vi "MPB_write_read_json text step array.vi"(8 "error in":errorcluster, 9 "json_array_from_file":T1[](array[typedef]) {"data num" format="%.3f"}, 10 "write_read":T3=enum."read", 11 "File Path":path) -> (0 "error out":errorcluster, 1 "steps array out":T1[](array[typedef]) {"data num" format="%.3f"}, 3 "File Path":path)   [LabVIEW 2020]
uses:
  controls/MPB_step.ctl
  controls/MPB_step_type.ctl
  controls/write_read.ctl
  3e47bdee-b09f-426d-96e8-78c270cf6aec.vi
  <vilib>/JDP Science/JSONtext/JSON text to Variant.vi
  <vilib>/JDP Science/JSONtext/JSONtext.lvlib
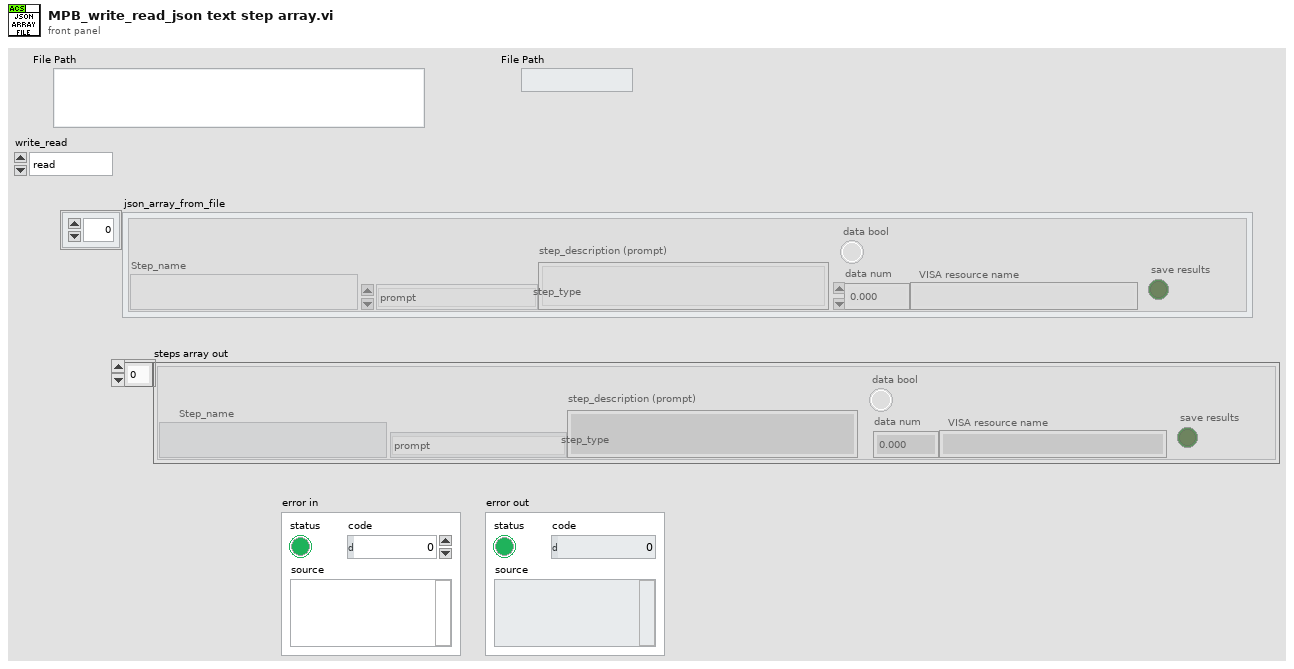
[diagram p1: front panel]
types:
  T1 = typedef "MPB_step.ctl" = cluster{"VISA resource name":string, "data num":dbl, "step_description (prompt)":string, "save results":bool, "step_type":T2, "Step_name":string, "data bool":bool}
  T2 = typedef "MPB_step_type.ctl" = enum16{"default", "prompt", "sequence#", "12V_1_power supply on_off", "12V_2_power supply on_off", "set_hipot_V", "set_hipot_I_limit", "set_hipot_ramping (sec)", "set hipot_hold_time", "read_hipot_V", "read_hipot_I", "set_daq", "read_daq", "flash uds", "wait (sec)", "record_pass_fail", "ac_charge_test", "dc_400V_charging", "HAPS Heater Output", "HAPS Compressor Output", "stop_test", "error_exit"}
  T3 = typedef "write_read.ctl" = enum16{"write", "read"}
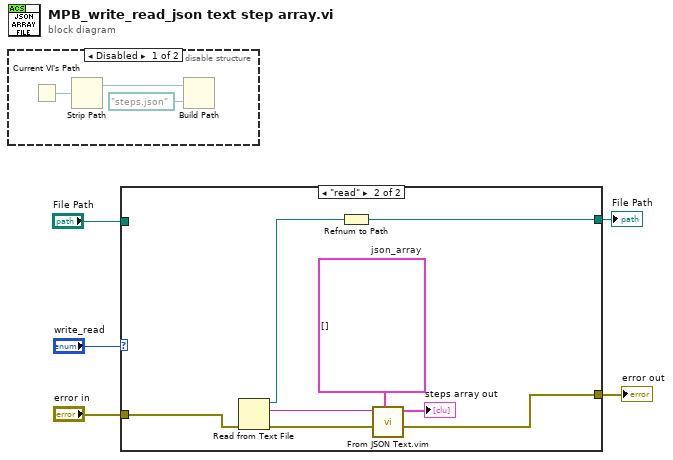
[diagram p0: block diagram]
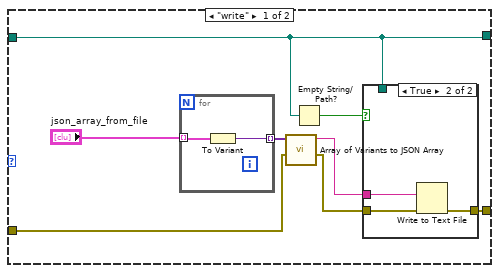
[diagram p3: hidden frame]
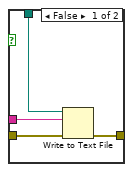
[diagram p4: hidden frame]
diagram:
  n1 = disable-structure shown="Disabled" {
    frame Disabled {
      n2 = Current VI's Path() -> (path=w8:path)
      n3 = Strip Path(path=w8) -> (stripped path=w7:path)  [unwired: 1 out]
      n4 = Build Path(base path=w7, name or relative path=path "steps.json") -> ()  [unwired: 1 out]
    }
    frame Enabled {
    }
  }
  n5 = case shown="\"read\"" "write_read" {
    tunnel: "error in" -> [w13 w30]
    tunnel: [w11 w28] -> w3
    tunnel: [w9 w26] -> w2
    tunnel: "File Path" -> [w9 _]
    frame "write" {
      n6 = for {
        tunnel: "json_array_from_file" -> [w24] mode=indexing
        tunnel: [w25] -> w16 mode=indexing
        n7 = To Variant(anything=w24) -> (Variant=w25:variant)
      }
      n8 = call <vilib>:"Array of Variants to JSON Array.vi"("error in (no error)"=w13, "Array of Variants"=w16) -> ("error out"=w12:errorcluster, "<JSON>"=w15:string)  [unwired: 8 in]
      n9 = Empty String/Path?(string/path=w9) -> (empty?=w10:bool)
      n10 = case shown="True" w10 {
        tunnel: w15 -> [w20 w23]
        tunnel: w12 -> [w19 w22]
        tunnel: [w18 w21] -> w11
        tunnel: w9 -> [w17 _]
        frame False {
          n11 = Write to Text File(file (use dialog)=w17, text=w20, error in=w19) -> (error out=w18:errorcluster)  [unwired: 1 in, 2 out]
        }
        frame True {
          n12 = Write to Text File(text=w23, error in=w22) -> (error out=w21:errorcluster)  [unwired: 2 in, 2 out]
        }
      }
    }
    frame "read" {
      w31 = T1[] []  # json_array
      n13 = Read from Text File(error in=w30) -> (refnum out=w27:refnum<file>, text=w32:string, error out=w29:errorcluster)  [unwired: 3 in, 1 out]
      n14 = Refnum to Path(1:w27) -> (0:w26:path)
      n15 = call "From JSON Text.vim"("Data Type and Default Value"=w31, "error in (no error)"=w29, "JSON"=w32) -> ("error out"=w28:errorcluster, "Data out"=→"steps array out":T1[])  [unwired: 7 in]
    }
  }
  "error out" <- w3
  "File Path" <- w2
